vi "Cleanup.vi"(8 "error in (no error)":errorcluster, 11 "Start Under Body Wash in":refnum<class "Start Under Body Wash.lvclass">) -> (0 "error out":errorcluster, 3 "Start Under Body Wash out":refnum<class "Start Under Body Wash.lvclass">)   [LabVIEW 2019, in "Start Under Body Wash.lvclass"]
uses:
  <vilib>/gpm_packages/@cs/Car-wash/Source/Process Steps/Start Under Body Wash/Start Under Body Wash.lvclass
  <vilib>/gpm_packages/@cs/Car-wash/Source/iProcess Step Model/iProcess Step Model/iProcess Step Model.lvclass
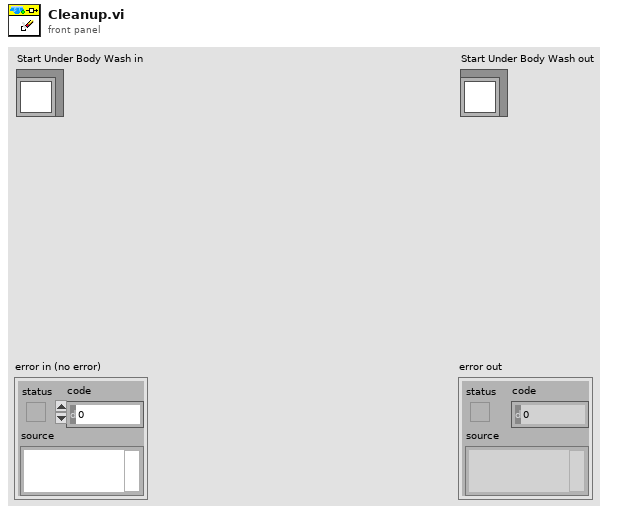
[diagram p1: front panel]
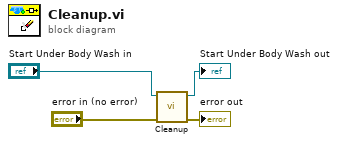
[diagram p0: block diagram]
diagram:
  n1 = call-parent "Cleanup.vi"("error in (no error)"="error in (no error)", "iProcess Step Model in"="Start Under Body Wash in") -> ("error out"=→"error out":errorcluster, "iProcess Step Model out"=→"Start Under Body Wash out":refnum<class "Start Under Body Wash.lvclass">)  [unwired: 8 in]
